vi "flow_event_init.vi"(11 "error in (no error)":errorcluster caption="エラー入力（エラーなし）") -> (4 "user_event":refnum<user-event>, 8 "event_refnum":refnum<event-registration>, 15 "error out":errorcluster caption="エラー出力")   [LabVIEW 2015]
uses:
  flow_queue_datatype.ctl
  flow_event_datatype.ctl
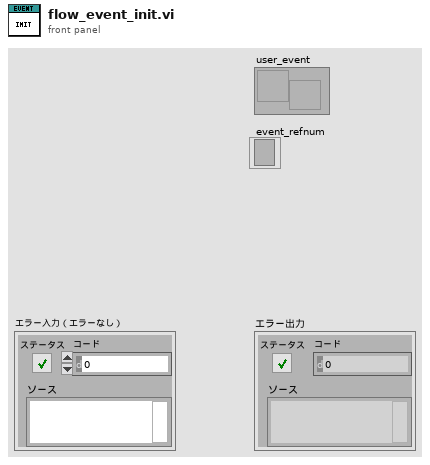
[diagram p1: front panel]
types:
  T1 = typedef "flow_event_datatype.ctl" = cluster{"command":string, "parameter":variant}
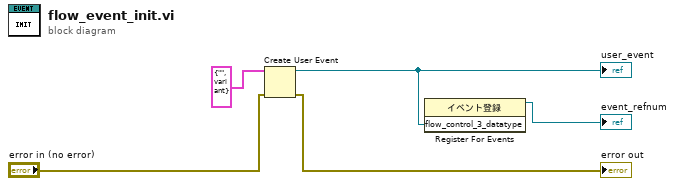
[diagram p0: block diagram]
diagram:
  n1 = Create User Event(user event datatype=T1 {"command"="", "parameter"=variant} ("flow_control_3_datatype"), error in="error in (no error)") -> (user event=w2:refnum<user-event>, error out=→"error out":errorcluster)
  "user_event" <- w2
  n2 = register-events(w2) -> (reference out=→"event_refnum":refnum<event-registration>)  [unwired: 2 in, 1 out]
